vi "SVL Calibrate Sensor (DAQmx).vi"(0 "DAQmx physical channel":tag, 1 "calibration settings":T9={"calibration value [EU rms]"=94.0, "calib. value is in dB"=TRUE, "calibration frequency [Hz]"=1000.0, "frequency tolerance [%]"=1.0} {"frequency tolerance [%]" format="%.2f"; "calibration value [EU rms]" format="%.2f"; "calibration frequency [Hz]" format="%.2f"}, 2 "channel configuration":T8={"maximum value (V)"=1.0, "minimum value (V)"=-1.0, "terminal configuration"=-1} {"terminal configuration" items=["Default"=-1, "RSE"=10083, "NRSE"=10078, "Differential"=10106, "Pseudodifferential"=12529]; "minimum value (V)" format="%.2f"; "maximum value (V)" format="%.2f"}, 3 "DSA channel settings":T7={"coupling"=10045, "enable IEPE excitation"=FALSE, "IEPE current [mA]"=2.0} {"IEPE current [mA]" format="%.1f"; "coupling" items=["AC"=10045, "DC"=10050, "GND"=10066]}, 4 "channel info":T10={"sensor sensitivity"=1000.0, "engineering units"=1, "dB reference"=1.0, "custom label"="EU", "weighting filter"=0, "pregain"=0.0} {"pregain" format="%.2f"; "weighting filter" items=["Linear", "A-weighting", "B-weighting", "C-weighting", "ITU-R 468-4", "Dolby", "CCITT", "C-message", "Wb", "Wc", "Wd", "We", "Wf", "Wh", "Wj", "Wk", "Wm", "AES17 20 kHz lowpass", "AES17 40 kHz lowpass", "AES17 20 kHz highpass", "AES17 40 kHz highpass"]; "dB reference" format="%^.1e"; "engineering units" items=["custom..."=0, "V"=1, "A"=21, "C"=30, "pC"=31, "s"=32, "-"=29, "Pa"=2, "N"=20, "g"=3, "m/s^2"=4, "m/s"=5, "m"=6, "mm/s"=12, "mm"=13, "micron/s"=14, "micron"=15, "in/s^2"=7, "in/s"=8, "in"=9, "mil/s"=10, "mil"=11, "rad/s^2"=16, "rad/s"=17, "rad"=18, "deg/s^2"=26, "deg/s"=27, "deg"=28, "RPM"=22, "cycle/s^2"=23, "Hz"=24, "cycle"=25, "strain"=19]; "sensor sensitivity" format="%#_5f"}, 5 "error in (no error)":errorcluster, 6 "sampling frequency [Hz]":dbl=50000.0 format="%.2f", 7 "self calibrate device (F)":bool, 8 "duration [s]":dbl=1.0 format="%.2f", 9 "time to settle [s]":dbl format="%_2f") -> (10 "power spectrum":cluster{"x0":dbl, "dx":dbl, "magnitude":dbl[]}(graph), 12 "spectrum info":T1={"channel name"="", "description"="", "x-axis units"=0, "spectral info"={"spectrum type"=enum."Power [Magnitude^2]", "linear/dB"=enum."linear", "window"=0, "window size"=0, "FFT size"=0}, "engineering units"=1, "custom label"="", "dB reference [EU]"=0.0, "peak units"=enum."rms", "weighting filter"=0, "spectral density?"=FALSE, "unit label"="", "spectrum skewed?"=FALSE, "complimentary spectrum units"=enum."none"} {"x-axis units" items=["Time (s)"=0, "Frequency-CB (Hz)"=1, "Frequency-CPB (Hz)"=1248, "Frequency-Arbitrary (Hz)"=2357, "Quefrency (s)"=2, "Revolutions (rev)"=3, "Order"=4, "Speed (RPM)"=11, "Speed (rad/s)"=21, "Index"=65535]; "weighting filter" items=["Linear", "A-weighting", "B-weighting", "C-weighting", "ITU-R 468-4", "Dolby", "CCITT", "C-message", "Wb", "Wc", "Wd", "We", "Wf", "Wh", "Wj", "Wk", "Wm", "AES17 20 kHz lowpass", "AES17 40 kHz lowpass", "AES17 20 kHz highpass", "AES17 40 kHz highpass"]; "dB reference [EU]" format="%.2f"; "engineering units" items=["custom..."=0, "V"=1, "A"=21, "C"=30, "pC"=31, "s"=32, "-"=29, "Pa"=2, "N"=20, "g"=3, "m/s^2"=4, "m/s"=5, "m"=6, "mm/s"=12, "mm"=13, "micron/s"=14, "micron"=15, "in/s^2"=7, "in/s"=8, "in"=9, "mil/s"=10, "mil"=11, "rad/s^2"=16, "rad/s"=17, "rad"=18, "deg/s^2"=26, "deg/s"=27, "deg"=28, "RPM"=22, "cycle/s^2"=23, "Hz"=24, "cycle"=25, "strain"=19]; "spectral info"."window" items=["None "=0, "Hanning"=1, "Hamming"=2, "Blackman-Harris"=3, "Exact Blackman"=4, "Blackman"=5, "Flat Top"=6, "4 Term B-Harris "=7, "7 Term B-Harris"=8, "Low Sidelobe"=9, "Force - Exponential"=10, "Gaussian"=62]}, 14 "calibrated sensor sensitivity [mV/EU]":dbl=1000.0 format="%.2f", 15 "calibrated channel info":T10={"sensor sensitivity"=1000.0, "engineering units"=1, "dB reference"=1.0, "custom label"="EU", "weighting filter"=0, "pregain"=0.0} {"pregain" format="%.2f"; "weighting filter" items=["Linear", "A-weighting", "B-weighting", "C-weighting", "ITU-R 468-4", "Dolby", "CCITT", "C-message", "Wb", "Wc", "Wd", "We", "Wf", "Wh", "Wj", "Wk", "Wm", "AES17 20 kHz lowpass", "AES17 40 kHz lowpass", "AES17 20 kHz highpass", "AES17 40 kHz highpass"]; "dB reference" format="%^.1e"; "engineering units" items=["custom..."=0, "V"=1, "A"=21, "C"=30, "pC"=31, "s"=32, "-"=29, "Pa"=2, "N"=20, "g"=3, "m/s^2"=4, "m/s"=5, "m"=6, "mm/s"=12, "mm"=13, "micron/s"=14, "micron"=15, "in/s^2"=7, "in/s"=8, "in"=9, "mil/s"=10, "mil"=11, "rad/s^2"=16, "rad/s"=17, "rad"=18, "deg/s^2"=26, "deg/s"=27, "deg"=28, "RPM"=22, "cycle/s^2"=23, "Hz"=24, "cycle"=25, "strain"=19]; "sensor sensitivity" format="%#_5f"}, 16 "amplitude [V rms]":dbl format="%.4f", 17 "frequency [Hz]":dbl format="%.2f", 19 "error out":errorcluster)   [LabVIEW 2017, in "SoundVib_Calibration.lvlib"]
doc: "Performs an end-to-end calibration on the selected channel by measuring the actual sensitivity of the sensor connected to the channel and returns the measured sensor sensitivity."
uses:
  <vilib>/addons/Sound and Vibration/svt_Calibration/SoundVib_Calibration.lvlib
  <vilib>/addons/_NISVFA/_Shared subVIs/Controls/svc_Channel Info.ctl
  <vilib>/addons/_NISVFA/_Shared subVIs/Controls/svc_Engineering Units Text Ring.ctl
  <vilib>/addons/_NISVFA/_Shared subVIs/Controls/svc_Weighting Filter Text Ring.ctl
  <vilib>/addons/_NISVFA/_Shared subVIs/Controls/svc_DSA Channel Settings.ctl
  <vilib>/addons/_NISVFA/_Shared subVIs/Controls/svc_Spectrum Info.ctl
  <vilib>/addons/_NISVFA/_Shared subVIs/Controls/svc_X-Axis Units.ctl
  <vilib>/addons/_NISVFA/_Shared subVIs/Controls/svc_Spectrum Type.ctl
  <vilib>/addons/_NISVFA/_Shared subVIs/Controls/svc_Complimentary Spectrum Units.ctl
  <vilib>/addons/_NISVFA/_Shared subVIs/Controls/svc_Window.ctl
  <vilib>/DAQmx/read.llb/DAQmx Read (Analog Wfm 1Chan NSamp).vi
  <vilib>/Utility/error.llb/Error Cluster From Error Code.vi
  <vilib>/addons/_NISVFA/_Spectrum Processing/SVFA Unit Conversion (Complex) (1 Ch).vi
  <vilib>/DAQmx/miscellaneous.llb/DAQmx Fill In Error Info.vi
  <vilib>/DAQmx/configure/timing.llb/DAQmx Timing (Sample Clock).vi
  <vilib>/DAQmx/create/channels.llb/DAQmx Create Channel (AI-Voltage-Basic).vi
  <vilib>/ErrorRing/Error Ring.xnode
  <resource>/objmgr/daqmx.rc
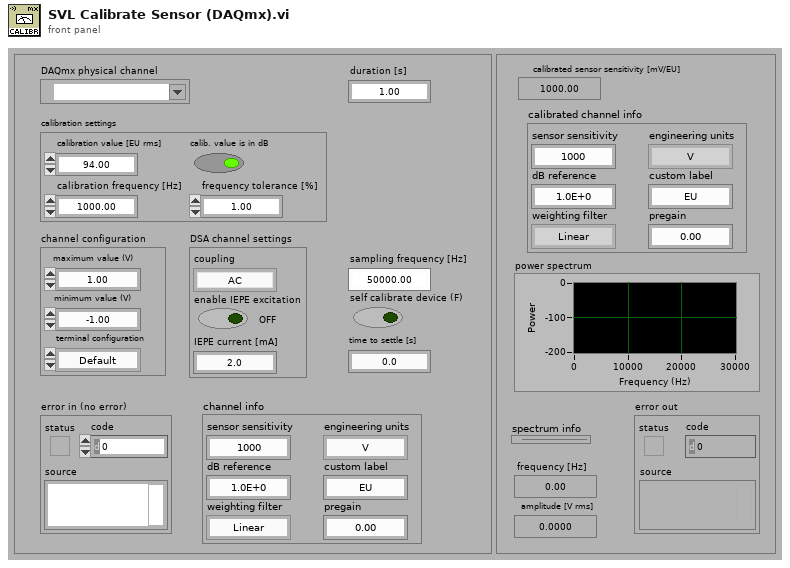
[diagram p1: front panel]
types:
  T1 = typedef "svc_Spectrum Info.ctl" = cluster{"channel name":string, "description":string, "x-axis units":T2, "spectral info":cluster{"spectrum type":T3, "linear/dB":enum16{"linear", "dB"}, "window":u16, "window size":i32, "FFT size":i32}, "engineering units":T4, "custom label":string, "dB reference [EU]":dbl, "peak units":enum16{"rms", "peak", "peak-peak"}, "weighting filter":T5, "spectral density?":bool, "unit label":string, "spectrum skewed?":bool, "complimentary spectrum units":T6}
  T2 = typedef "svc_X-Axis Units.ctl" = u16
  T3 = typedef "svc_Spectrum Type.ctl" = enum16{"FFT Spectrum [complex]", "Amplitude [Magnitude]", "Power [Magnitude^2]", "Cross Spectrum [complex]", "Frequency Response [Complex]"}
  T4 = typedef "svc_Engineering Units Text Ring.ctl" = u16
  T5 = typedef "svc_Weighting Filter Text Ring.ctl" = u16
  T6 = typedef "svc_Complimentary Spectrum Units.ctl" = enum16{"none", "radians", "degrees", "cycles", "imaginary"}
  T7 = typedef "svc_DSA Channel Settings.ctl" = cluster{"coupling":i32, "enable IEPE excitation":bool, "IEPE current [mA]":dbl}
  T8 = cluster{"maximum value (V)":dbl, "minimum value (V)":dbl, "terminal configuration":i32}
  T9 = cluster{"calibration value [EU rms]":dbl, "calib. value is in dB":bool, "calibration frequency [Hz]":dbl, "frequency tolerance [%]":dbl}
  T10 = typedef "svc_Channel Info.ctl" = cluster{"sensor sensitivity":dbl, "engineering units":T4, "dB reference":dbl, "custom label":string, "weighting filter":T5, "pregain":dbl}
  T11 = cluster{"linear/dB":enum16{"no change", "linear", "dB"}, "dB reference":dbl, "power/magnitude":enum16{"no change", "power", "magnitude"}, "view":enum16{"no change", "rms", "peak", "peak-peak"}}
  T12 = enum16{"none", "input signal", "detected signal", "residual signal"}
  T13 = typedef "svc_Window.ctl" = u32
  T14 = cluster{"complex spectrum response":cluster{"f0":dbl, "df":dbl, "complex spectrum":cdb[]}, "spectrum info":T1}
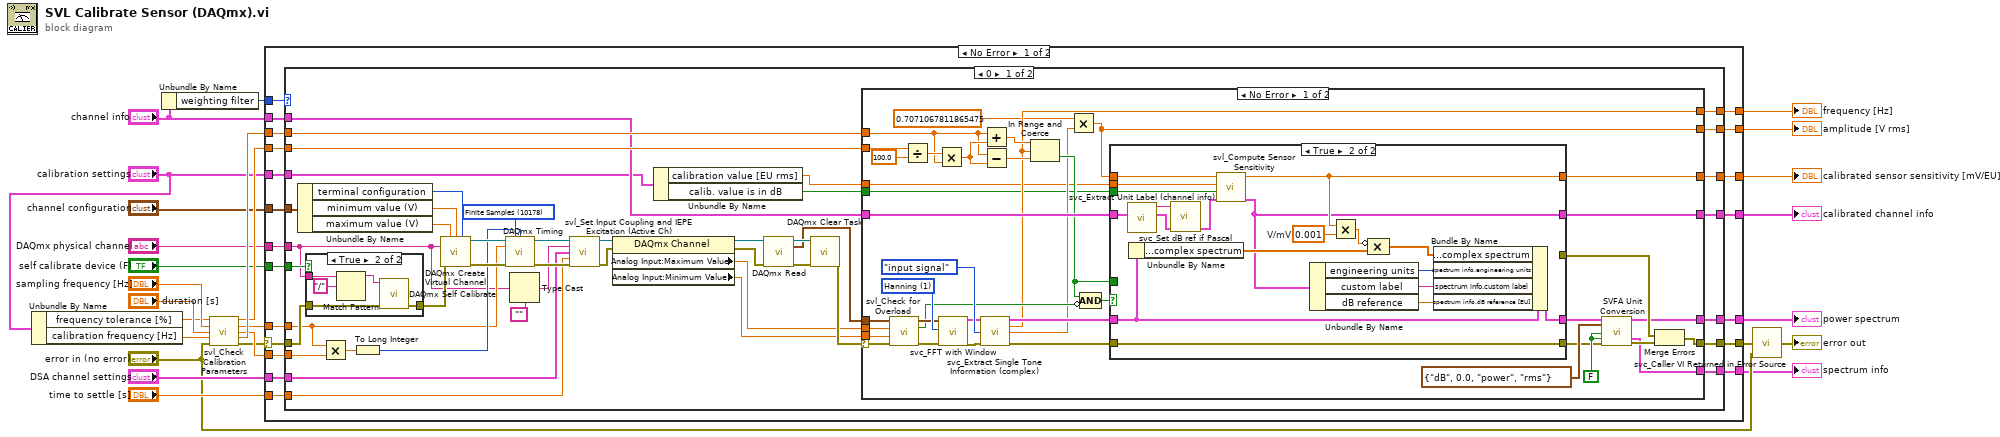
[diagram p0: block diagram]
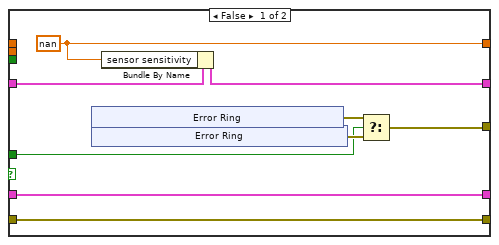
[diagram p3: hidden frame]
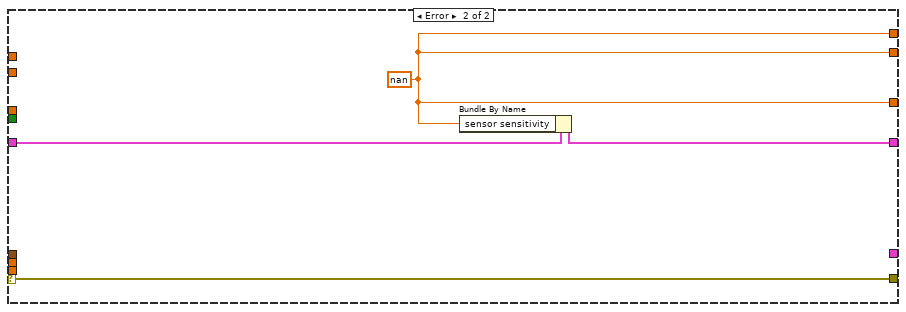
[diagram p4: hidden frame]
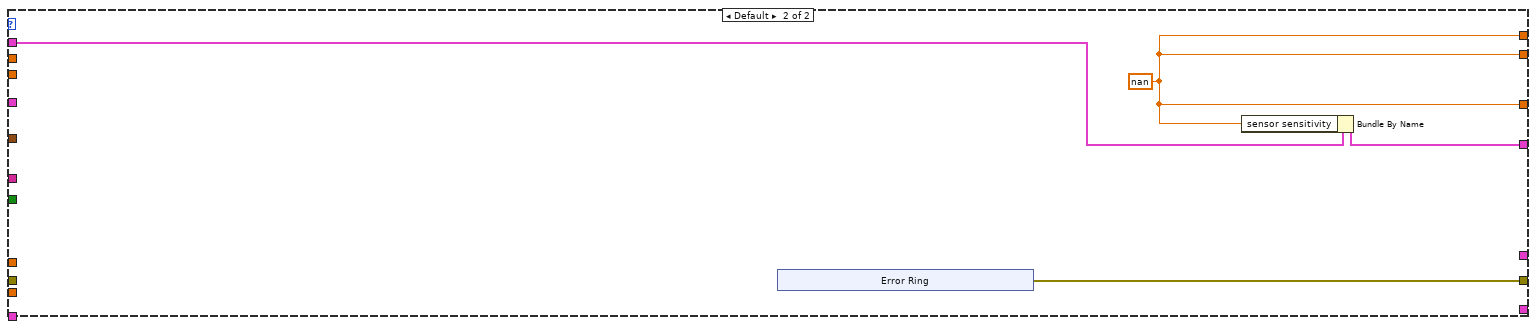
[diagram p5: hidden frame]
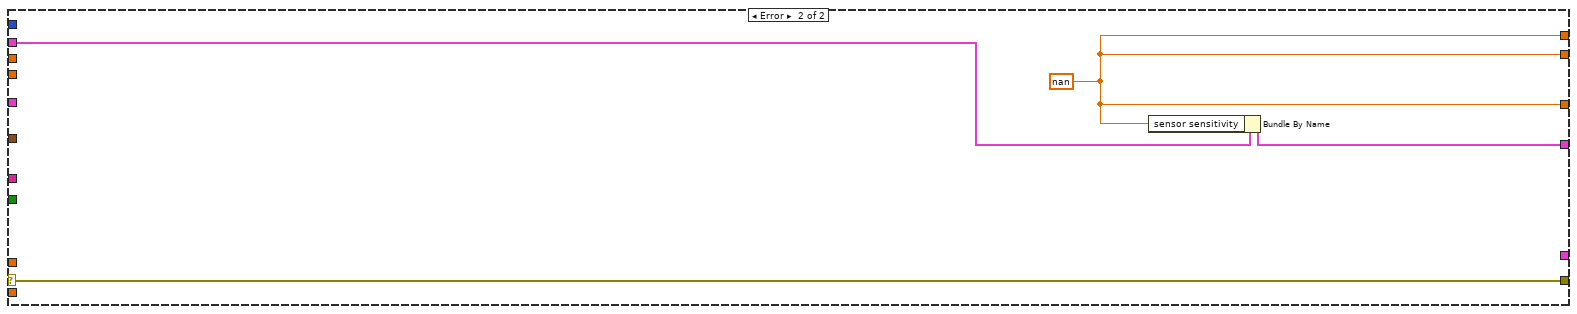
[diagram p6: hidden frame]
diagram:
  n1 = Unbundle By Name("calibration settings") -> ("frequency tolerance [%]"=w11:dbl, "calibration frequency [Hz]"=w6:dbl)
  n2 = Unbundle By Name("channel info") -> ("weighting filter"=w1:T5)
  n3 = call <vilib>:"svl_Check Calibration Parameters.vi"("frequency tolerance [%]"=w11, "sampling frequency [Hz]"="sampling frequency [Hz]", "duration [s]"="duration [s]", "calibration frequency [Hz]"=w6, "error in (no error)"="error in (no error)") -> ("dup frequency tolerance [%]"=w19:dbl, "dup sampling frequency [Hz]"=w18:dbl, "dup duration [s]"=w15:dbl, "dup calibration frequency [Hz]"=w20:dbl, "error out"=w14:errorcluster)  [unwired: 6 in]
  n4 = case shown="No Error" w14 {
    selector: w14 -> [w33 w188]
    tunnel: w18 -> [w46 _]
    tunnel: w15 -> [w45 _]
    tunnel: [w44 w187] -> w26
    tunnel: [w43 w187] -> w25
    tunnel: [w42 w185] -> w22
    tunnel: [w41 w187] -> w24
    tunnel: [w40 w188] -> w23
    tunnel: "self calibrate device (F)" -> [w39 _]
    tunnel: "channel info" -> [w38 w186]
    tunnel: w1 -> [w37 _]
    tunnel: w20 -> [w36 _]
    tunnel: w19 -> [w35 _]
    tunnel: "DAQmx physical channel" -> [w34 _]
    tunnel: "channel configuration" -> [w32 _]
    tunnel: "DSA channel settings" -> [w31 _]
    tunnel: "calibration settings" -> [w30 _]
    tunnel: "time to settle [s]" -> [w29 _]
    tunnel: [w28 _] -> w4
    tunnel: [w27 _] -> w3
    frame No Error {
      n5 = case shown="0" w37 {
        tunnel: w46 -> [w60 _]
        tunnel: w45 -> [w90 _]
        tunnel: [w89 w179] -> w44
        tunnel: [w88 w179] -> w43
        tunnel: [w87 w177] -> w42
        tunnel: [w86 w179] -> w41
        tunnel: w38 -> [w58 w178]
        tunnel: [w85 w180] -> w40
        tunnel: w39 -> [w84 _]
        tunnel: w36 -> [w83 _]
        tunnel: w35 -> [w82 _]
        tunnel: w34 -> [w50 _]
        tunnel: w33 -> [w81 _]
        tunnel: w32 -> [w64 _]
        tunnel: w31 -> [w63 _]
        tunnel: w30 -> [w49 _]
        tunnel: w29 -> [w62 _]
        tunnel: [w53 _] -> w28
        tunnel: [w52 _] -> w27
        frame 0 {
          w78 = 10178 items=["Finite Samples"=10178, "Continuous Samples"=10123] ("sample mode")
          n6 = Unbundle By Name(w64) -> ("terminal configuration"=w74:i32, "minimum value (V)"=w75:dbl, "maximum value (V)"=w76:dbl)
          n7 = case shown="True" w84 {
            tunnel: w81 -> [w91 w96]
            tunnel: [w91 w95] -> w65
            tunnel: w50 -> [_ w92]
            frame False {
            }
            frame True {
              n8 = Match Pattern(string=w92, regular expression="/") -> (before substring=w93:string)  [unwired: 1 in, 3 out]
              n9 = call <vilib>:"DAQmx Self Calibrate.vi"("device in"=w93, "error in"=w96) -> ("error out"=w95:errorcluster)  [unwired: 13 in]
            }
          }
          n10 = Multiply(x=w60, y=w90) -> (x*y=w80:dbl)
          n11 = To Long Integer(number=w80) -> (32bit integer=w61:i32)
          n12 = call-poly <vilib>:"DAQmx Create Virtual Channel.vi"("maximum value"=w76, "minimum value"=w75, "input terminal configuration"=w74, "physical channels"=w50, "error in"=w65) -> ("task out"=w71:refnum<k21>, "error out"=w68:errorcluster)  [unwired: 9 in]
          n13 = call-poly <vilib>:"DAQmx Timing.vi"("task/channels in"=w71, "sample mode"=w78, "samples per channel"=w61, "rate"=w60, "error in"=w68) -> ("task out"=w70:refnum<k21>, "error out"=w67:errorcluster)  [unwired: 9 in]
          n14 = Type Cast(type="", x=w50) -> (*(type *) &x=w54:string)
          n15 = call <vilib>:"svl_Set Input Coupling and IEPE Excitation (Active Ch).vi"("AI task name"=w70, "active channels"=w54, "DSA channel settings"=w63, "time to settle [s]"=w62, "error in (no error)"=w67) -> ("dup AI task name"=w73:refnum<k21>, "error out"=w72:errorcluster)  [unwired: 9 in]
          n16 = property class="DAQmx Channel"(reference=w73, error in=w72) -> (reference out=w69:refnum<k21>, error out=w66:errorcluster, "Analog Input:Maximum Value"=w56:dbl, "Analog Input:Minimum Value"=w57:dbl)
          n17 = Unbundle By Name(w49) -> ("calibration value [EU rms]"=w48:dbl, "calib. value is in dB"=w47:bool)
          n18 = call-poly <vilib>:"DAQmx Read.vi"("task/channels in"=w69, "error in"=w66) -> ("task out"=w79:refnum<k21>, "data"=w51:waveform(dbl), "error out"=w77:errorcluster)  [unwired: 11 in]
          n19 = call <vilib>:"DAQmx Clear Task.vi"("task in"=w79, "error in"=w77) -> ("error out"=w59:errorcluster)  [unwired: 13 in]
          n20 = case shown="No Error" w59 {
            selector: w59 -> [w133 w176]
            tunnel: [w112 w174] -> w89
            tunnel: [w136 w174] -> w88
            tunnel: [w135 w173] -> w87
            tunnel: [w113 w174] -> w86
            tunnel: w58 -> [w134 w175]
            tunnel: [w103 w176] -> w85
            tunnel: w83 -> [w117 _]
            tunnel: w82 -> [w118 _]
            tunnel: w51 -> [w132 _]
            tunnel: w57 -> [w131 _]
            tunnel: w56 -> [w130 _]
            tunnel: [w102 _] -> w53
            tunnel: [w101 _] -> w52
            tunnel: w48 -> [w98 _]
            tunnel: w47 -> [w97 _]
            frame No Error {
              w110 = FALSE ("convert to degree (T)")
              w124 = T13 1 items=["None ", "Hanning", "Hamming", "Blackman-Harris", "Exact Blackman", "Blackman", "Flat Top", "4 Term B-Harris ", "7 Term B-Harris", "Low Sidelobe", "Force - Exponential", "Gaussian"] ("window")
              n21 = call <vilib>:"svl_Check for Overload.vi"("error in (no error)"=w133, "minimum input value (V)"=w131, "maximum input value (V)"=w130, "signal [V]"=w132) -> ("error out"=w120:errorcluster, "overload"=w115:bool, "dup signal [V]"=w121:waveform(dbl))  [unwired: 5 in]
              n22 = Divide(x=w118, y=100.0) -> (x/y=w126:dbl)
              n23 = Multiply(x=w126, y=w117) -> (x*y=w127:dbl)
              n24 = call <vilib>:"svc_FFT with Window.vi"("time signal in [EU]"=w121, "window"=w124, "error in (no error)"=w120) -> ("complex spectrum"=w122:T14, "error out"=w100:errorcluster)  [unwired: 15 in]
              n25 = call <vilib>:"svc_Extract Single Tone Information (complex).vi"("complex spectrum"=w122, "export signals"=T12."input signal", "error in"=w100) -> ("complex spectrum"=w119:T14, "frequency [Hz]"=w113:dbl, "amplitude [EU pk]"=w107:dbl, "error out"=w99:errorcluster)  [unwired: 7 in, 2 out]
              n26 = Add(x=w117, y=w127) -> (x+y=w128:dbl)
              n27 = Subtract(x=w117, y=w127) -> (x-y=w129:dbl)
              n28 = In Range and Coerce(upper limit=w128, x=w113, lower limit=w129) -> (In Range?=w116:bool)  [unwired: 1 out]
              n29 = Multiply(x=0.7071067811865475 ("sqrt(x)"), y=w107) -> (x*y=w112:dbl)
              n30 = Compound Arithmetic op=AND(w116, invert w115) -> (w114:bool)
              n31 = case shown="True" w114 {
                tunnel: [w143 w171] -> w136
                tunnel: [w145 w157] -> w135
                tunnel: w134 -> [w144 w172]
                tunnel: w99 -> [w138 w154]
                tunnel: [w137 w160] -> w109
                tunnel: w119 -> [w137 w165]
                tunnel: w112 -> [_ w164]
                tunnel: w116 -> [w140 _]
                tunnel: [w139 _] -> w106
                tunnel: [w138 w154] -> w105
                tunnel: w98 -> [_ w156]
                tunnel: w97 -> [_ w155]
                frame False {
                  w143 = nan ("est frequency peak")
                  n32 = xnode "Error Ring"() -> ("error out"=w142:errorcluster)
                  n33 = xnode "Error Ring"() -> ("error out"=w141:errorcluster)
                  n34 = Bundle By Name(cluster=w144, "sensor sensitivity"=w143) -> (w145:T10)
                  n35 = Select(t=w142, s=w140, f=w141) -> (s? t:f=w139:errorcluster)
                }
                frame True {
                  w170 = 0.001  # V/mV
                  n36 = call <vilib>:"svc_Extract Unit Label (channel info).vi"("channel info"=w172) -> ("channel info"=w162:T10, "unit label"=w161:string)  [unwired: 8 in, 1 out]
                  n37 = Unbundle By Name(w165) -> ("complex spectrum response.complex spectrum"=w159:cdb[])
                  n38 = call <vilib>:"svc_Set dB ref if Pascal.vi"("channel info"=w162, "unit label"=w161) -> ("channel info"=w163:T10)  [unwired: 4 in, 1 out]
                  n39 = call <vilib>:"svl_Compute Sensor Sensitivity.vi"("channel info in"=w163, "calib. value is in dB (F)"=w155, "calibration value [EUrms]"=w156, "amplitude (Vrms)"=w164) -> ("channel info out"=w157:T10, "sensor sensitivity [mV/EU]"=w171:dbl)  [unwired: 6 in]
                  n40 = Unbundle By Name(w157) -> ("engineering units"=w168:T4, "custom label"=w167:string, "dB reference"=w166:dbl)
                  n41 = Multiply(x=w171, y=w170) -> (x*y=w169:dbl)
                  n42 = Compound Arithmetic op=MULTIPLY(invert w169, w159) -> (w158:cdb[])
                  n43 = Bundle By Name(cluster=w165, "complex spectrum response.complex spectrum"=w158, "spectrum info.engineering units"=w168, "spectrum info.custom label"=w167, "spectrum info.dB reference [EU]"=w166) -> (w160:T14)
                }
              }
              n44 = call-poly <vilib>:"SVFA Unit Conversion.vi"("complex spectrum"=w109, "desired scaling"=T11 {"linear/dB"=enum."dB", "dB reference"=0.0, "power/magnitude"=enum."power", "view"=enum."rms"}, "unwrap phase (F)"=w110, "convert to degree (T)"=w110, "error in (no error)"=w105) -> ("converted spectrum"=w102:cluster{"x0":dbl, "dx":dbl, "magnitude":dbl[]}, "spectrum info out"=w101:T1, "error out"=w104:errorcluster)  [unwired: 9 in, 3 out]
              n45 = Merge Errors(w106, w104) -> (w103:errorcluster)
            }
            frame Error {
              w174 = nan
              n46 = Bundle By Name(cluster=w175, "sensor sensitivity"=w174) -> (w173:T10)
            }
          }
        }
        frame Default {
          w179 = nan ("sensor sensitivity [mV/EU]")
          n47 = xnode "Error Ring"() -> ("error out"=w180:errorcluster)
          n48 = Bundle By Name(cluster=w178, "sensor sensitivity"=w179) -> (w177:T10)
        }
      }
    }
    frame Error {
      w187 = nan ("sensor sensitivity [mV/EU]")
      n49 = Bundle By Name(cluster=w186, "sensor sensitivity"=w187) -> (w185:T10)
    }
  }
  "amplitude [V rms]" <- w26
  "calibrated sensor sensitivity [mV/EU]" <- w25
  "frequency [Hz]" <- w24
  "calibrated channel info" <- w22
  "power spectrum" <- w4
  "spectrum info" <- w3
  n50 = call <vilib>:"svc_Caller VI Returned in Error Source.vi"("warning input to caller"="error in (no error)", "error in (no error)"=w23) -> ("error out"=→"error out":errorcluster)  [unwired: 3 in]
